vi "Distance Test.vi"(9 "Cluster":T1={"Parameter 1"=0.0, "Parameter 2"=0.0, "Camera view angle"=30.7} {"Camera view angle" format="%#_13g"}, 10 "Rectangle":T2, 11 "Y Image Resolution":i32) -> (2 "Distance (in)":dbl)   [LabVIEW 2013]
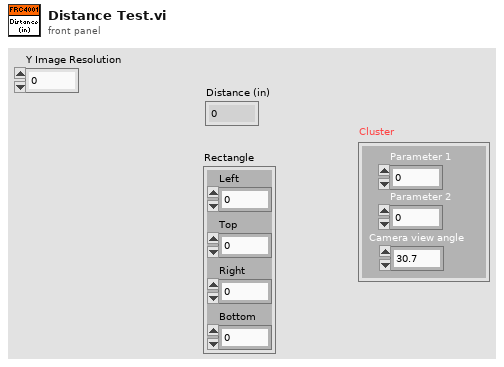
[diagram p1: front panel]
types:
  T1 = cluster{"Parameter 1":dbl, "Parameter 2":dbl, "Camera view angle":dbl}
  T2 = cluster{"Left":dbl, "Top":dbl, "Right":dbl, "Bottom":dbl}
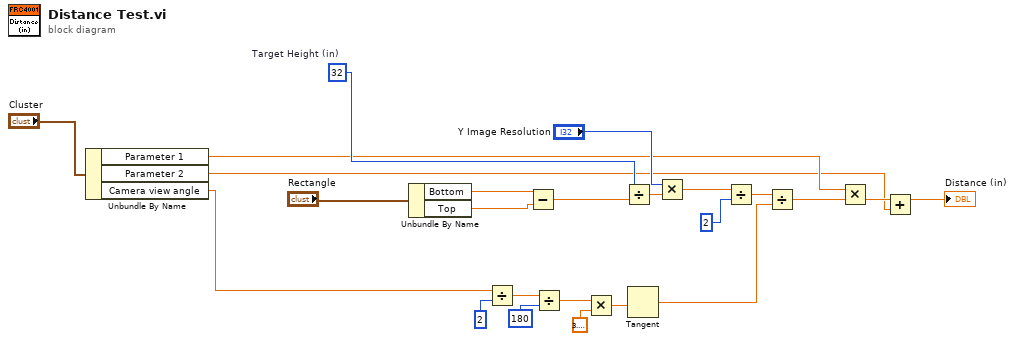
[diagram p0: block diagram]
diagram:
  w7 = 32  # Target Height (in)
  n1 = Unbundle By Name("Cluster") -> ("Parameter 1"=w3:dbl, "Parameter 2"=w2:dbl, "Camera view angle"=w1:dbl)
  n2 = Unbundle By Name("Rectangle") -> ("Bottom"=w13:dbl, "Top"=w12:dbl)
  n3 = Divide(x=w1, y=2) -> (x/y=w17:dbl)
  n4 = Subtract(x=w13, y=w12) -> (x-y=w11:dbl)
  n5 = Divide(x=w17, y=180) -> (x/y=w18:dbl)
  n6 = Multiply(x=w18, y=3.141592653589793) -> (x*y=w16:dbl)
  n7 = Divide(x=w7, y=w11) -> (x/y=w20:dbl)
  n8 = Tangent(1:w16) -> (0:w24:dbl)
  n9 = Multiply(x="Y Image Resolution", y=w20) -> (x*y=w10:dbl)
  n10 = Divide(x=w10, y=2) -> (x/y=w23:dbl)
  n11 = Divide(x=w23, y=w24) -> (x/y=w8:dbl)
  n12 = Multiply(x=w3, y=w8) -> (x*y=w6:dbl)
  n13 = Add(x=w6, y=w2) -> (x+y=→"Distance (in)":dbl)
